vi "update-timeseries-plots.vi"(8 "error in (no error)":errorcluster, 10 "input cluster":T1, 11 "data-in":dbl[][](array[numeric])) -> (0 "error out":errorcluster)   [LabVIEW 2017]
uses:
  controls/scan-plots-timeseries.ctl
  controls/time-series-graph-ref.ctl
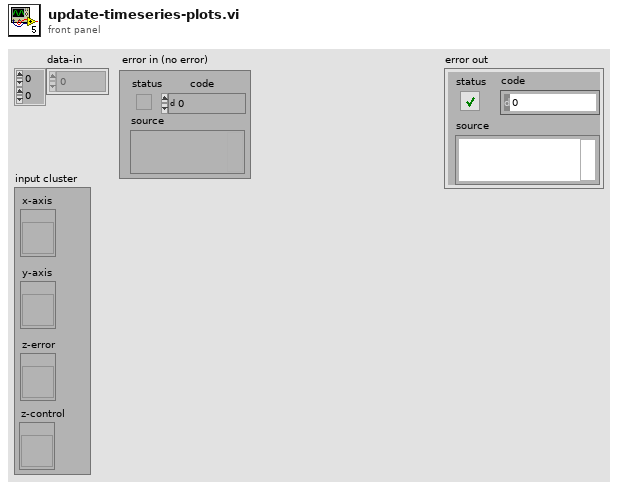
[diagram p1: front panel]
types:
  T1 = typedef "scan-plots-timeseries.ctl" = cluster{"x-axis":T2, "y-axis":T2, "z-error":T2, "z-control":T2}
  T2 = typedef "time-series-graph-ref.ctl" = refnum<vi>
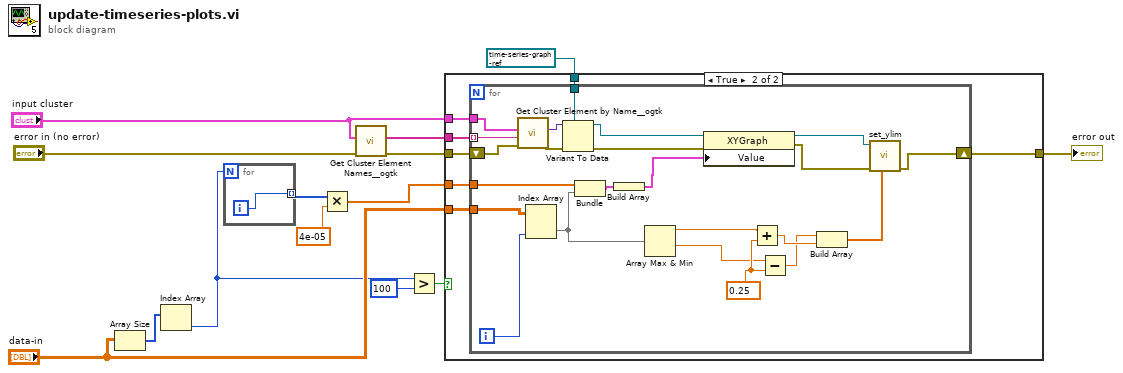
[diagram p0: block diagram]
diagram:
  n1 = Array Size(array="data-in") -> (size(s)=w6:i32[])
  n2 = Index Array(array=w6) -> (element=w2:i32)  [unwired: 1 in]
  n3 = for {
    N: w2 -> [_]
    tunnel: [w15] -> w10 mode=indexing
    i -> [w15]
  }
  n4 = Multiply(x=w10, y=4e-05) -> (x*y=w8:dbl[])
  n5 = call <userlib>:"Get Cluster Element Names__ogtk.vi"("error in (no error)"="error in (no error)", "Cluster"="input cluster") -> ("error out"=w12:errorcluster, "Element Names"=w14:string[])  [unwired: 8 in]
  n6 = Greater?(x=w2, y=100) -> (0:w3:bool)
  n7 = case shown="True" w3 {
    tunnel: w14 -> [_ w23]
    tunnel: "input cluster" -> [_ w22]
    tunnel: w12 -> [w16 w21]
    tunnel: T2 refnum ("signal-select") -> [_ w20]
    tunnel: w8 -> [_ w19]
    tunnel: "data-in" -> [_ w18]
    tunnel: [w16 w17] -> w4
    frame False {
    }
    frame True {
      n8 = for {
        tunnel: w23 -> [w45] mode=indexing
        tunnel: w22 -> [w46]
        shift-right: [w24] -> w17
        shift-left: w21 -> [w44]
        tunnel: w20 -> [w40]
        tunnel: w18 -> [w38]
        tunnel: w19 -> [w36]
        i -> [w37]
        w31 = 0.25
        n9 = call <userlib>:"Get Cluster Element by Name__ogtk.vi"("error in (no error)"=w44, "Element Name"=w45, "Cluster"=w46) -> ("error out"=w43:errorcluster, "VElement"=w41:variant)  [unwired: 6 in, 1 out]
        n10 = Index Array(array=w38, index (col)=w37) -> (element=w26:dbl[])  [unwired: 1 in]
        n11 = Variant To Data(error in=w43, type=w40, Variant=w41) -> (data=w39:T2, error out=w42:errorcluster)
        n12 = Bundle(w36, "data-in"=w26) -> (w35:cluster{dbl[], "data-in":dbl[]})  [unwired: 1 in]
        n13 = Build Array(w35) -> (w34:cluster{dbl[], "data-in":dbl[]}[])
        n14 = Array Max & Min(array=w26) -> (max value=w29:dbl, min value=w30:dbl)  [unwired: 2 out]
        n15 = property on="Property Node" class="XYGraph"(reference=w39, error in=w42, "Value"=w34) -> (reference out=w33:T2, error out=w32:errorcluster)
        n16 = Add(x=w29, y=w31) -> (x+y=w28:dbl)
        n17 = Subtract(x=w30, y=w31) -> (x-y=w27:dbl)
        n18 = Build Array(w27, w28) -> (w25:dbl[])
        n19 = call "set_ylim.vi"("ylim"=w25, "error in"=w32, "figure (in)"=w33) -> ("error out"=w24:errorcluster)  [unwired: 7 in, 1 out]
      }
    }
  }
  "error out" <- w4
